vi "CalculateSwerveDriveDistance.vi"(11 "Actual Pivot System":T1) -> (0 "error out":errorcluster, 3 "Total Distance (in)":dbl)   [LabVIEW 2019]
uses:
  Controls/Robot Pivot Motion Commands.ctl
  Controls/Pivot Motor Commands.ctl
  Controls/Robot Drive Mode.ctl
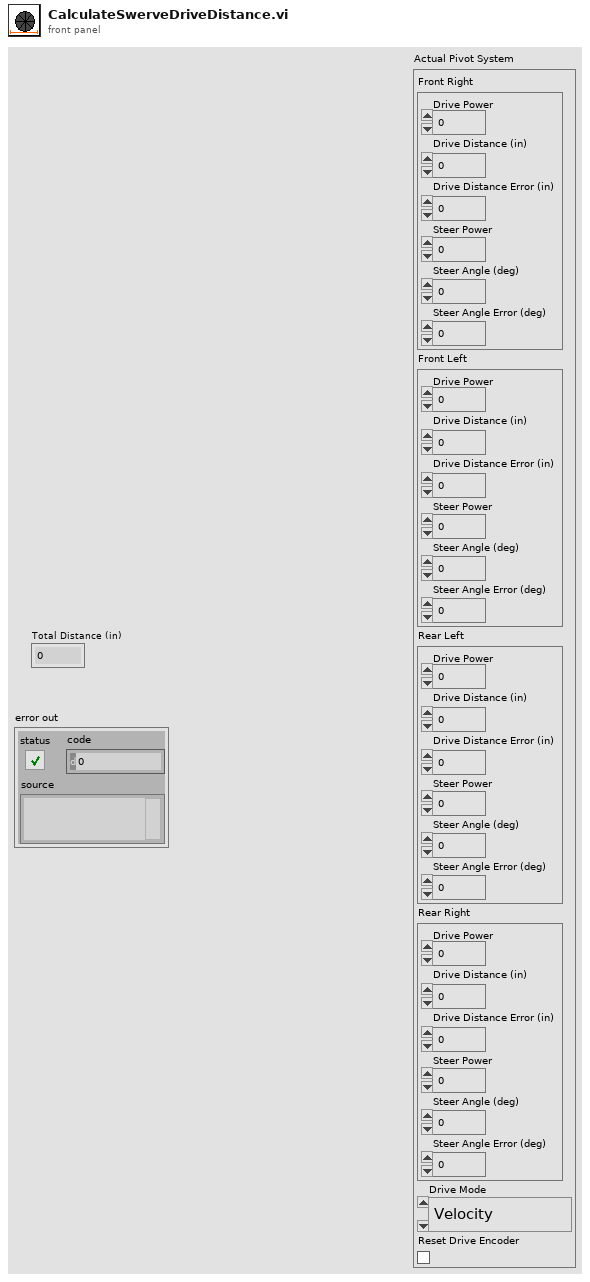
[diagram p1: front panel]
types:
  T1 = typedef "Robot Pivot Motion Commands.ctl" = cluster{"Front Right":T2, "Front Left":T2, "Rear Left":T2, "Rear Right":T2, "Drive Mode":T3, "Reset Drive Encoder":bool}
  T2 = typedef "Pivot Motor Commands.ctl" = cluster{"Drive Power":dbl, "Drive Distance (in)":dbl, "Drive Distance Error (in)":dbl, "Steer Power":dbl, "Steer Angle (deg)":dbl, "Steer Angle Error (deg)":dbl}
  T3 = typedef "Robot Drive Mode.ctl" = enum16{"Velocity", "Distance"}
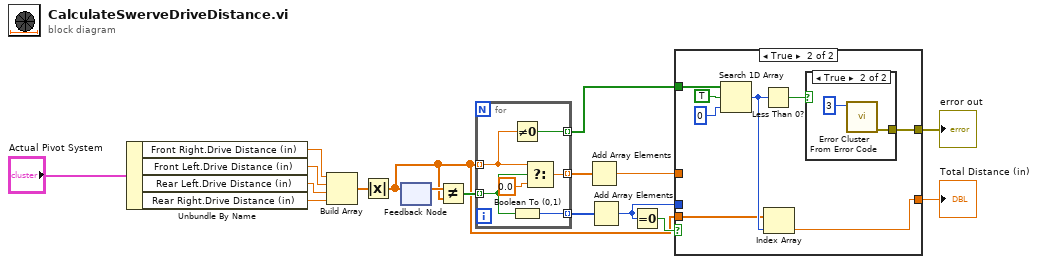
[diagram p0: block diagram]
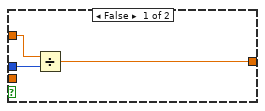
[diagram p2: hidden frame]
diagram:
  n1 = Unbundle By Name("Actual Pivot System") -> ("Front Right.Drive Distance (in)"=w9:dbl, "Front Left.Drive Distance (in)"=w15:dbl, "Rear Left.Drive Distance (in)"=w14:dbl, "Rear Right.Drive Distance (in)"=w13:dbl)
  n2 = Build Array(w9, w15, w14, w13) -> (w12:dbl[])
  n3 = Absolute Value(x=w12) -> (abs(x)=w1:dbl[])
  n4 = feedback #1() -> (w16:dbl[])  [unwired: 1 in]
  n5 = feedback-in #1(w1) -> ()
  n6 = Not Equal?(x=w16, y=w1) -> (x != y?=w7:bool[])
  n7 = for {
    tunnel: w7 -> [w22] mode=indexing
    tunnel: w1 -> [w19] mode=indexing
    tunnel: [w21] -> w11 mode=indexing
    tunnel: [w20] -> w8 mode=indexing
    tunnel: [w18] -> w2 mode=indexing
    n8 = Not Equal To 0?(x=w19) -> (x != 0?=w18:bool)
    n9 = Boolean To (0,1)(Boolean=w22) -> (0, 1=w21:i16)
    n10 = Select(t=w19, s=w22, f=0.0) -> (s? t:f=w20:dbl)
  }
  n11 = Add Array Elements(numeric array=w8) -> (sum=w4:dbl)
  n12 = Add Array Elements(numeric array=w11) -> (sum=w3:i16)
  n13 = Equal To 0?(x=w3) -> (x = 0?=w10:bool)
  n14 = case shown="True" w10 {
    tunnel: w1 -> [_ w28]
    tunnel: [w24 w27] -> w6
    tunnel: [_ w34] -> w5
    tunnel: w4 -> [w26 _]
    tunnel: w3 -> [w25 _]
    tunnel: w2 -> [_ w33]
    frame False {
      n15 = Divide(x=w26, y=w25) -> (x/y=w24:dbl)
    }
    frame True {
      n16 = Search 1D Array(1D array=w33, element=TRUE, start index (0)=0) -> (index of element=w29:i32)
      n17 = Less Than 0?(x=w29) -> (x < 0?=w30:bool)
      n18 = Index Array(array=w28, index=w29) -> (element=w27:dbl)
      n19 = case shown="True" w30 {
        tunnel: [_ w36] -> w34
        frame False {
        }
        frame True {
          n20 = call <vilib>:"Error Cluster From Error Code.vi"("error code (0)"=3) -> ("error out"=w36:errorcluster)  [unwired: 8 in]
        }
      }
    }
  }
  "Total Distance (in)" <- w6
  "error out" <- w5
